vi "N6701A_ReadCurrentStandalone.vi"(8 "error in (no error)":errorcluster, 10 "Channel Name (1)":string="2", 11 "VISA resource name":refnum<visa-resource-name>="PS2") -> (0 "error out":errorcluster, 2 "Measurement":dbl=-0.0009589195 format="%^.3e")   [LabVIEW 2015]
uses:
  <instrlib>/Agilent N6700 Series/Agilent N6700 Series.lvlib
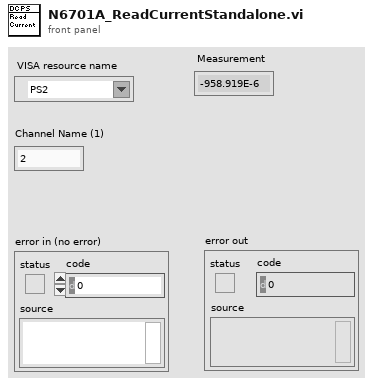
[diagram p1: front panel]
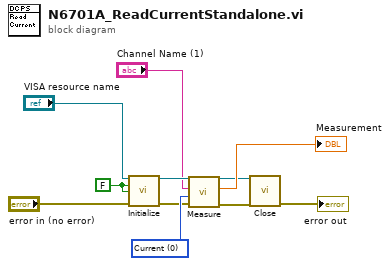
[diagram p0: block diagram]
diagram:
  w4 = FALSE ("ID Query? (T: Yes)")
  w10 = 0 items=["Voltage"=1, "Current"=0] ("Measurement Type (1: Voltage)")
  n1 = call <instrlib>:"Initialize.vi"("VISA resource name"="VISA resource name", "ID Query? (T: Yes)"=w4, "Reset? (T: Yes)"=w4, "error in (no error)"="error in (no error)") -> ("VISA resource name out"=w9:refnum<visa-resource-name>, "error out"=w8:errorcluster)  [unwired: 10 in]
  n2 = call <instrlib>:"Measure.vi"("error in (no error)"=w8, "Measurement Type (1: Voltage)"=w10, "Channel Name (1)"="Channel Name (1)", "VISA resource name"=w9) -> ("error out"=w3:errorcluster, "Measurement"=→"Measurement":dbl, "VISA resource name out"=w2:refnum<visa-resource-name>)  [unwired: 5 in]
  n3 = call <instrlib>:"Close.vi"("VISA resource name"=w2, "error in (no error)"=w3) -> ("error out"=→"error out":errorcluster)  [unwired: 13 in]
